vi "SRV_Manage Time Interval for Read.vi"(9 "Some State":bool, 12 "Read Interval (1000 ms)":u32=1000) -> (8 "Time to Read?":bool, 10 "State Change?":bool)   [LabVIEW 2014]
doc: "Returns True only after Read Interval milliseconds have passed since the last time a true was returned.\n\n\nAuthor: Mike Schultz - Logic PD"
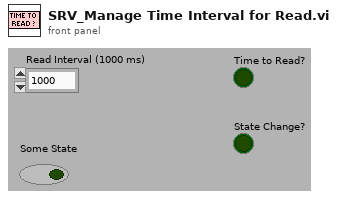
[diagram p1: front panel]
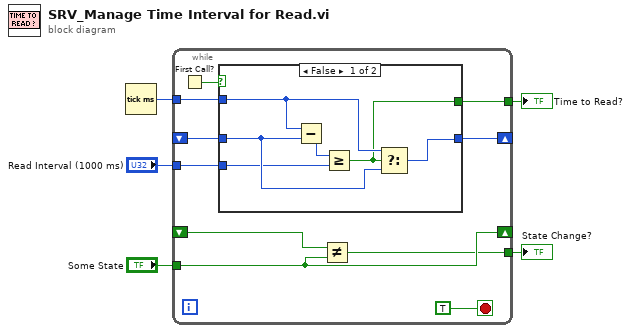
[diagram p0: block diagram]
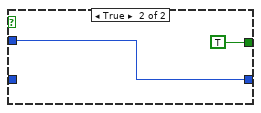
[diagram p2: hidden frame]
diagram:
  n1 = Tick Count (ms)() -> (millisecond timer value=w5:u32)
  n2 = while {
    shift-right: [w13] -> _
    shift-left: _ -> [w12]
    tunnel: w5 -> [w14]
    tunnel: [w10] -> w2
    tunnel: "Read Interval (1000 ms)" -> [w9]
    shift-right: [w7] -> _
    shift-left: _ -> [w8]
    tunnel: "Some State" -> [w7]
    tunnel: [w6] -> w1
    stop <- TRUE stop-if-true
    n3 = First Call?() -> (First Call?: T/F=w11:bool)
    n4 = case shown="False" w11 {
      tunnel: w14 -> [w20 w22]
      tunnel: [w19 w22] -> w13
      tunnel: w12 -> [w18 _]
      tunnel: [w17 TRUE] -> w10
      tunnel: w9 -> [w16 _]
      frame False {
        n5 = Subtract(x=w20, y=w18) -> (x-y=w21:u32)
        n6 = Greater Or Equal?(x=w21, y=w16) -> (x >= y?=w17:bool)
        n7 = Select(t=w20, s=w17, f=w18) -> (s? t:f=w19:u32)
      }
      frame True {
      }
    }
    n8 = Not Equal?(x=w8, y=w7) -> (x != y?=w6:bool)
  }
  "Time to Read?" <- w2
  "State Change?" <- w1
